vi "Post (NT).vi"(7 "PV name":string, 8 "error in (no error)":errorcluster, 10 "value in":refnum<class "NT Base.lvclass">, 11 "Server in":refnum<class "Server.lvclass">) -> (0 "error out":errorcluster, 2 "value out":refnum<class "NT Base.lvclass">, 3 "Server out":refnum<class "Server.lvclass">)   [LabVIEW 2020, in "PV Access.lvlib" / "PVA Server.lvlib" / "Server.lvclass"]
uses:
  Server.lvclass/Server.ctl
  Server.lvclass
  Source/Source.lvclass
  PV Data/NT Base/NT Base.lvclass
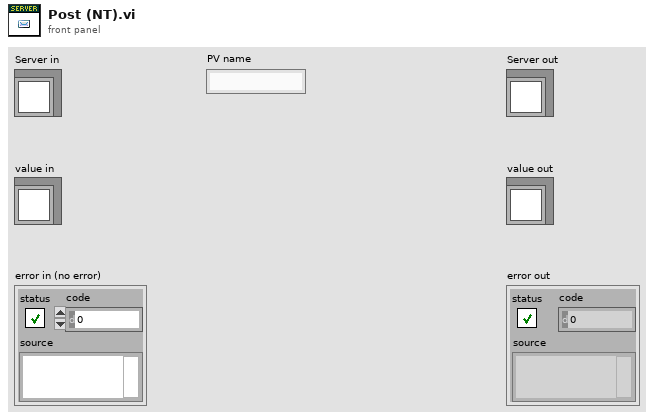
[diagram p1: front panel]
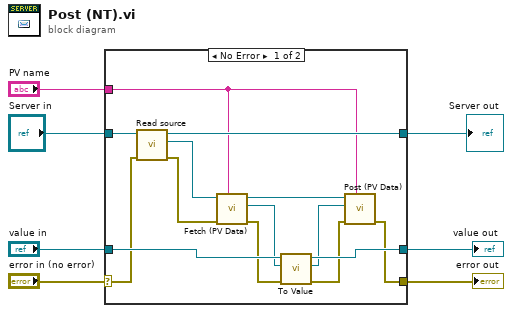
[diagram p0: block diagram]
diagram:
  n1 = case shown="No Error" "error in (no error)" {
    selector: "error in (no error)" -> [w14 w24]
    tunnel: [w15 w24] -> w4
    tunnel: [w20 w23] -> w3
    tunnel: "Server in" -> [w21 w23]
    tunnel: "PV name" -> [w16 _]
    tunnel: "value in" -> [w18 w22]
    tunnel: [w19 w22] -> w1
    frame No Error {
      n2 = call "Read source.vi"("error in (no error)"=w14, "Server in"=w21) -> ("error out"=w13:errorcluster, "Source"=w17:refnum<class "Source.lvclass">, "Server out"=w20:refnum<class "Server.lvclass">)  [unwired: 7 in]
      n3 = call "Fetch (PV Data).vi"("PV name"=w16, "error in"=w13, "Source in"=w17) -> ("error out"=w10:errorcluster, "PV Data out"=w9:refnum<class "PV Data.lvclass">, "Source out"=w12:refnum<class "Source.lvclass">)  [unwired: 6 in]
      n4 = call-dynamic "To Value.vi"("error in (no error)"=w10, "PV Data in"=w9, "NT Base in"=w18) -> ("error out"=w11:errorcluster, "PV Data out"=w8:refnum<class "PV Data.lvclass">, "NT Base out"=w19:refnum<class "NT Base.lvclass">)  [unwired: 6 in]
      n5 = call "Post (PV Data).vi"("PV name"=w16, "error in"=w11, "PV Data in"=w8, "Source in"=w12) -> ("error out"=w15:errorcluster)  [unwired: 6 in, 1 out]
    }
    frame Error {
    }
  }
  "error out" <- w4
  "Server out" <- w3
  "value out" <- w1
